vi "Cmd New.vi"(4 "error in (no error)":errorcluster, 5 "mode (create new)":T1(ring), 6 "initial data":T2, 7 "object name (unnamed)":string) -> (0 "error out":errorcluster, 1 "status":enum16{"error", "new object", "existing object"}(ring), 3 "command reference":T4)   [LabVIEW 2020, in "NI_Database_API.lvlib"]
doc: "Looks up an existing <B>Command</B> object matching <B>object name</B> or creates a new Command object and returns a refnum you can use when calling other Command methods.\n\n<B>mode</B> specify whether you want to <B>create</B> a new object or <B>lookup</B> an existing object.\n\n<B>status</B> returns whether a new or an existing object reference is returned.\n\nObjects created with this VI should be destroyed using the <B>Command Delete</B> VI."
uses:
  <vilib>/addons/database/NI_Database_API.lvlib
  <vilib>/addons/database/Command.llb/Cmd ObjectReference.ctl
  <vilib>/addons/database/Command.llb/Cmd DataMembers.ctl
  <vilib>/addons/database/Connection.llb/Conn ObjectReference.ctl
  <vilib>/Utility/_goopsup.llb/GOOP Object Repository Method.ctl
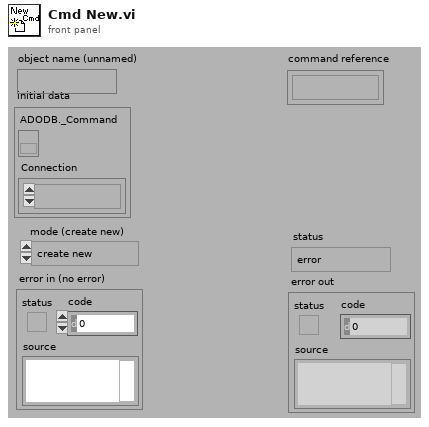
[diagram p1: front panel]
types:
  T1 = enum16{"create new", "lookup existing", "lookup or create"}
  T2 = typedef "NI_Database_API.lvlib/Cmd DataMembers.ctl" = cluster{"ADODB._Command":refnum<k7>, "Connection":T3}
  T3 = typedef "NI_Database_API.lvlib/Conn ObjectReference.ctl" = refnum<k1>
  T4 = typedef "NI_Database_API.lvlib/Cmd ObjectReference.ctl" = refnum<k1>
  T5 = typedef "GOOP Object Repository Method.ctl" = enum16{"Create", "GetCopy", "GetModify", "Set", "Destroy", "Create Static", "Get All Refs", "Reset", "Get Statistics"}
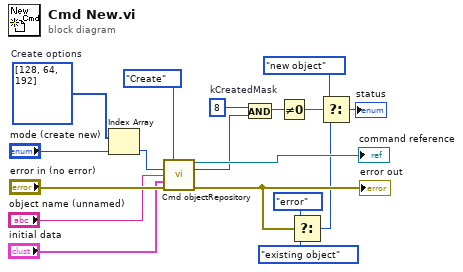
[diagram p0: block diagram]
diagram:
  w9 = i32[] [128, 64, 192]  # Create options
  w12 = 8  # kCreatedMask
  n1 = Index Array(array=w9, index="mode (create new)") -> (element=w8:i32)
  n2 = call <vilib>:"Cmd objectRepository.vi"("method"=GOOP_Object_Repository_Method."Create", "flags in"=w8, "name in"="object name (unnamed)", "classDataIn"="initial data", "error in (no error)"="error in (no error)") -> ("command reference out"=→"command reference":T4, "flags out"=w11:i32, "error out"=w18:errorcluster)  [unwired: 4 in, 4 out]
  "error out" <- w18
  n3 = And(x=w12, y=w11) -> (x .and. y?=w7:i32)
  n4 = Not Equal To 0?(x=w7) -> (x != 0?=w6:bool)
  n5 = Select(t=enum16{"error", "new object", "existing object"}."error" ("status"), s=w18, f=enum16{"error", "new object", "existing object"}."existing object" ("status")) -> (s? t:f=w2:enum16{"error", "new object", "existing object"})
  n6 = Select(t=enum16{"error", "new object", "existing object"}."new object" ("status"), s=w6, f=w2) -> (s? t:f=→"status":enum16{"error", "new object", "existing object"})
